vi "Setup.vi"(8 "Error In":errorcluster, 11 "Address":string) -> (0 "Error Out":errorcluster, 2 "Known Host":refnum<class "Known Host.lvclass">, 3 "Known Hosts":refnum<class "Known Hosts.lvclass">)   [LabVIEW 2018, in "Tests.lvlib" / "Known Host.lvlib"]
uses:
  Known Host.lvlib
  src/Toolkit/Known Hosts/Known Hosts.lvclass
  src/Toolkit/Known Host/Known Host.lvclass
  <vilib>/Utility/error.llb/Clear Errors.vi
  <vilib>/Utility/sysdir.llb/Get System Directory.vi
  src/Toolkit/Known Host/Support/Create from Known Hosts.vi
  src/Toolkit/SSH/SSH.lvclass
  src/Toolkit/Session/Session.lvclass
  Tests.lvlib
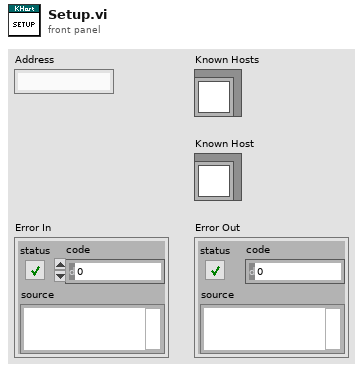
[diagram p1: front panel]
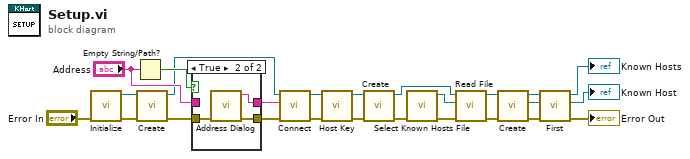
[diagram p0: block diagram]
diagram:
  n1 = call "Initialize.vi"("Error In"="Error In") -> ("Error Out"=w18:errorcluster, "SSH"=w7:refnum<class "SSH.lvclass">)  [unwired: 9 in]
  n2 = Empty String/Path?(string/path="Address") -> (empty?=w21:bool)
  n3 = call "Create.vi"("Error In"=w18, "SSH"=w7) -> ("Error Out"=w23:errorcluster, "Sesssion"=w20:refnum<class "Session.lvclass">)  [unwired: 8 in]
  n4 = case shown="True" w21 {
    tunnel: w23 -> [w26 w30]
    tunnel: [w26 w29] -> w24
    tunnel: [w27 w28] -> w25
    tunnel: "Address" -> [w27 _]
    frame False {
    }
    frame True {
      n5 = call "Address Dialog.vi"("Error In"=w30) -> ("Error Out"=w29:errorcluster, "Address Out"=w28:string)  [unwired: 9 in]
    }
  }
  n6 = call "Connect.vi"("Error In"=w24, "Address"=w25, "Session In"=w20) -> ("Error Out"=w16:errorcluster, "Sesssion Out"=w17:refnum<class "Session.lvclass">)  [unwired: 7 in]
  n7 = call "Host Key.vi"("Error In"=w16, "Session In"=w17) -> ("Error Out"=w15:errorcluster, "Sesssion Out"=w10:refnum<class "Session.lvclass">)  [unwired: 6 in, 2 out]
  n8 = call "Create.vi"("Error In"=w15, "Session"=w10) -> ("Error Out"=w14:errorcluster, "Known Hosts"=w12:refnum<class "Known Hosts.lvclass">)  [unwired: 8 in]
  n9 = call "Select Known Hosts File.vi"("Error In"=w14) -> ("Error Out"=w13:errorcluster, "Known Hosts File"=w11:path)  [unwired: 9 in]
  n10 = call "Read File.vi"("Error In"=w13, "File"=w11, "KnownHosts In"=w12) -> ("Error Out"=w9:errorcluster, "KnownHosts Out"=w3:refnum<class "Known Hosts.lvclass">)  [unwired: 6 in, 1 out]
  n11 = call-poly "Create.vi"("Error In"=w9, "Known Hosts In"=w3) -> ("Error Out"=w8:errorcluster, "Known Host"=w1:refnum<class "Known Host.lvclass">, "Known Hosts Out"=w2:refnum<class "Known Hosts.lvclass">)  [unwired: 7 in]
  n12 = call "First.vi"("Error In"=w8, "Known Host In"=w1, "KnownHosts In"=w2) -> ("Error Out"=→"Error Out":errorcluster, "Known Host Out"=→"Known Host":refnum<class "Known Host.lvclass">, "KnownHosts Out"=→"Known Hosts":refnum<class "Known Hosts.lvclass">)  [unwired: 5 in, 1 out]
